vi "Main.vi"   [LabVIEW 2017, in "Builder Pattern Demo.lvclass"]
uses:
  Builder Pattern Demo.lvclass
  Meal Builder Class/MealBuilder.lvclass
  Meal Class/Meal.lvclass
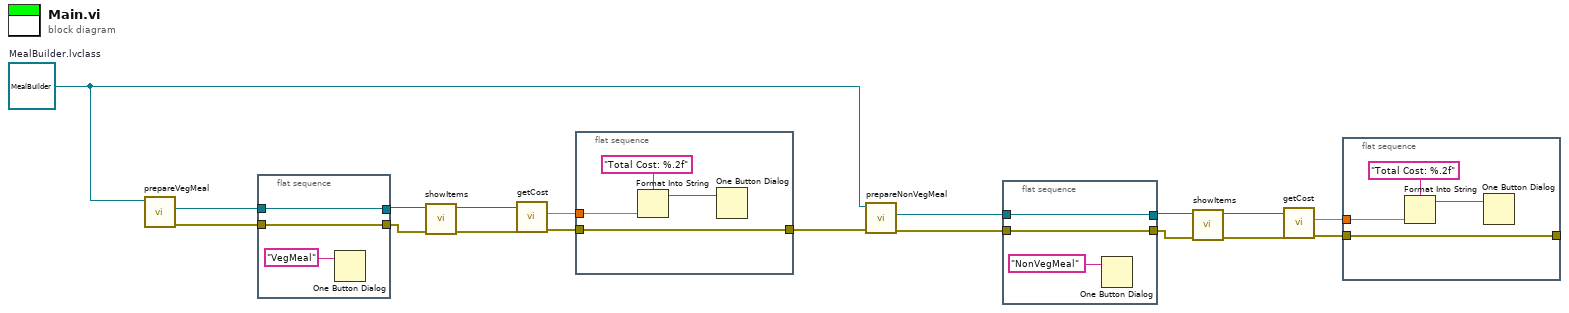
[diagram p0: block diagram]
diagram:
  w2 = refnum<class "MealBuilder.lvclass"> refnum  # MealBuilder.lvclass
  n1 = call-dynamic "prepareVegMeal.vi"("MealBuilder in"=w2) -> ("error out"=w15:errorcluster, "Meal out"=w1:refnum<class "Meal.lvclass">)  [unwired: 8 in, 1 out]
  n2 = flat-sequence {
    tunnel: [w20] -> w18
    tunnel: w1 -> [w20]
    tunnel: w15 -> [w19]
    tunnel: [w19] -> w14
    frame #0 {
      n3 = One Button Dialog(message="VegMeal") -> ()  [unwired: 1 in, 1 out]
    }
  }
  n4 = call-dynamic "showItems.vi"("error in (no error)"=w14, "Meal in"=w18) -> ("error out"=w13:errorcluster, "Meal out"=w17:refnum<class "Meal.lvclass">)  [unwired: 8 in]
  n5 = call-dynamic "getCost.vi"("error in (no error)"=w13, "Meal in"=w17) -> ("error out"=w12:errorcluster, "cost"=w16:dbl)  [unwired: 7 in, 1 out]
  n6 = flat-sequence {
    tunnel: w16 -> [w23]
    tunnel: [w22] -> w3
    tunnel: w12 -> [w22]
    frame #0 {
      n7 = Format Into String(format string="Total Cost: %.2f", w23) -> (resulting string=w24:string)  [unwired: 2 in, 1 out]
      n8 = One Button Dialog(message=w24) -> ()  [unwired: 1 in, 1 out]
    }
  }
  n9 = call-dynamic "prepareNonVegMeal.vi"("error in (no error)"=w3, "MealBuilder in"=w2) -> ("error out"=w8:errorcluster, "Meal out"=w4:refnum<class "Meal.lvclass">)  [unwired: 7 in, 1 out]
  n10 = flat-sequence {
    tunnel: [w27] -> w5
    tunnel: w4 -> [w27]
    tunnel: w8 -> [w26]
    tunnel: [w26] -> w9
    frame #0 {
      n11 = One Button Dialog(message="NonVegMeal") -> ()  [unwired: 1 in, 1 out]
    }
  }
  n12 = call-dynamic "showItems.vi"("error in (no error)"=w9, "Meal in"=w5) -> ("error out"=w10:errorcluster, "Meal out"=w6:refnum<class "Meal.lvclass">)  [unwired: 8 in]
  n13 = call-dynamic "getCost.vi"("error in (no error)"=w10, "Meal in"=w6) -> ("error out"=w11:errorcluster, "cost"=w7:dbl)  [unwired: 7 in, 1 out]
  n14 = flat-sequence {
    tunnel: w7 -> [w30]
    tunnel: [w29] -> _
    tunnel: w11 -> [w29]
    frame #0 {
      n15 = Format Into String(format string="Total Cost: %.2f", w30) -> (resulting string=w31:string)  [unwired: 2 in, 1 out]
      n16 = One Button Dialog(message=w31) -> ()  [unwired: 1 in, 1 out]
    }
  }
